vi "asset.attach_dataset_add_tag.vi"(8 "error in":errorcluster, 11 "AssetAttachDatasetStaging in":refnum<class "AssetAttachDatasetStaging.lvclass">) -> (0 "error out":errorcluster, 3 "AssetAttachDatasetStaging out":refnum<class "AssetAttachDatasetStaging.lvclass">)   [LabVIEW 2020, in "AssetAttachDatasetStaging.lvclass"]
doc: "Adds a series-tag filter to the dataset attachment being staged."
uses:
  AssetAttachDatasetStaging.lvclass
  AssetAttachDatasetStaging.lvclass/AssetAttachDatasetStaging.ctl
  client.lvlib
panel:
  in  "key":string
  in  "value":string
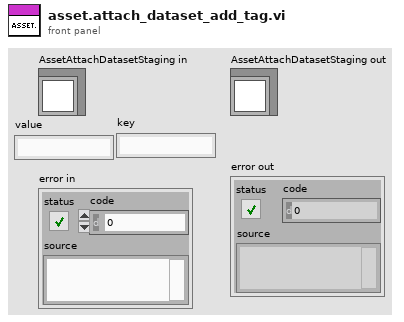
[diagram p1: front panel]
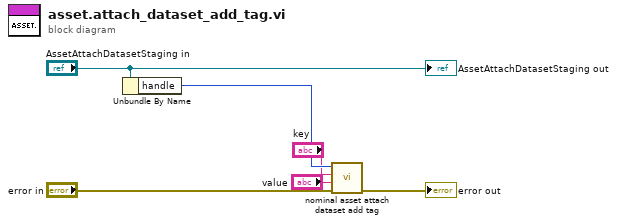
[diagram p0: block diagram]
diagram:
  n1 = Unbundle By Name("AssetAttachDatasetStaging in") -> ("handle"=w4:i32)
  n2 = call "nominal asset attach dataset add tag.vi"("error in (no error)"="error in", "value"="value", "key"="key", "staging"=w4) -> ("error out"=→"error out":errorcluster)  [unwired: 6 in, 1 out]
  "AssetAttachDatasetStaging out" <- "AssetAttachDatasetStaging in"
